vi "Levenberg Marquardt P.D.vi"(0 "x":dbl format="%.2f", 1 "A":dbl[](array[numeric]) format="%.2f", 2 "variable":i32[](array[numeric]), 3 "result":dbl[](array[numeric]) format="%.2f", 4 "table":i32[][](array[numeric])) -> (5 "dy(y,a)/da":dbl[](array[numeric]) format="%.2f")   [LabVIEW 2017, in "NI_Gmath.lvlib"]
uses:
  NI_Gmath.lvlib
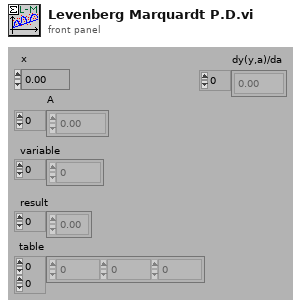
[diagram p1: front panel]
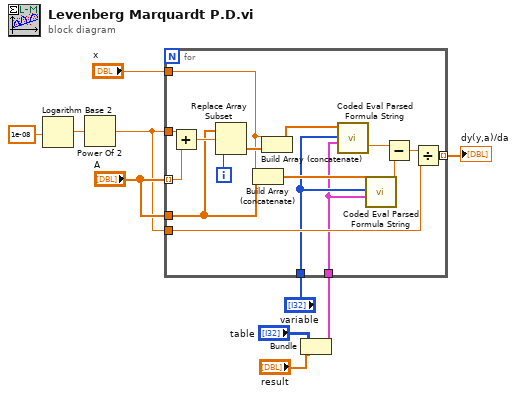
[diagram p0: block diagram]
diagram:
  n1 = Logarithm Base 2(1:1e-08) -> (0:w7:dbl)
  n2 = Power Of 2(x=w7) -> (2^x=w6:dbl)
  n3 = Bundle("table"="table", "result"="result") -> (w1:cluster{"table":i32[][], "result":dbl[]})  [unwired: 1 in]
  n4 = for {
    tunnel: w6 -> [w26]
    tunnel: "A" -> [w25] mode=indexing
    tunnel: "x" -> [w16]
    tunnel: "A" -> [w18]
    tunnel: w6 -> [w21]
    tunnel: [w20] -> w8 mode=indexing
    tunnel: "variable" -> [w12]
    tunnel: w1 -> [w11]
    i -> [w23]
    n5 = Add(x=w26, y=w25) -> (x+y=w24:dbl)
    n6 = Replace Array Subset(array=w18, new element=w24, index=w23) -> (w17:dbl[])
    n7 = Build Array (concatenate)(w16, w18) -> (w14:dbl[])
    n8 = Build Array (concatenate)(w16, w17) -> (w13:dbl[])
    n9 = call "Coded Eval Parsed Formula String.vi"("Parsed Formula"=w11, "Variables"=w12, "X Values"=w13) -> ("y value"=w15:dbl)  [unwired: 1 in, 1 out]
    n10 = call "Coded Eval Parsed Formula String.vi"("Parsed Formula"=w11, "Variables"=w12, "X Values"=w14) -> ("y value"=w19:dbl)  [unwired: 1 in, 1 out]
    n11 = Subtract(x=w15, y=w19) -> (x-y=w22:dbl)
    n12 = Divide(x=w22, y=w21) -> (x/y=w20:dbl)
  }
  "dy(y,a)/da" <- w8
